vi "LVCAM Msg Receive.vi"(11 "Self Actor in":refnum<class "Self Actor.lvclass">) -> (1 "DeQ Msg?":bool, 2 "Msg":refnum<class "Msg.lvclass">)   [LabVIEW 2021, in "LVCAM.lvlib" / "Self Actor.lvclass"]
uses:
  Self Actor.lvclass
  Msg/Msg.lvclass
  Self Actor.lvclass/Self Actor.ctl
  Msgs/LVCAM Nest Destroyed/LVCAM Nest Destroyed Msg/LVCAM Nest Destroyed Msg.lvclass
  C:/PPLs/LabVIEW-Composed-Actor-Model-LVCAM/LabVIEW-Composed-Actor-Model-LVCAM/AAM/LVCAM/Msg/Msg.lvclass
  Msgs/LVCAM Destroy Self/LVCAM Destroy Self Msg/LVCAM Destroy Self Msg.lvclass
  Msg Q/Msg Q.lvclass
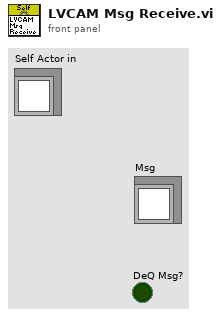
[diagram p1: front panel]
types:
  T1 = typedef "LVCAM.lvlib/Self Actor.lvclass/State.ctl" = enum16{"Safe Msging", "Destroying Self"}
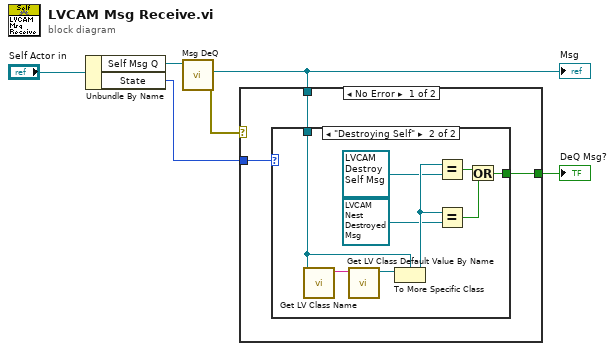
[diagram p0: block diagram]
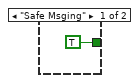
[diagram p2: hidden frame]
diagram:
  n1 = Unbundle By Name("Self Actor in") -> ("Self Msg Q"=w5:refnum<class "Msg Q.lvclass">, "State"=w3:T1)
  n2 = call "Msg DeQ.vi"("Msg Queue in"=w5) -> ("error out"=w6:errorcluster, "Msg"=w1:refnum<class "Msg.lvclass">)  [unwired: 9 in]
  "Msg" <- w1
  n3 = case shown="No Error" w6 {
    tunnel: w1 -> [w7 _]
    tunnel: [w8 _] -> w4
    tunnel: w3 -> [w9 _]
    frame No Error {
      n4 = case shown="\"Destroying Self\"" w9 {
        tunnel: w7 -> [_ w16]
        tunnel: [TRUE w13] -> w8
        frame "Safe Msging" {
        }
        frame "Destroying Self" {
          n5 = call <vilib>:"Get LV Class Name.vi"("object"=w16) -> ("class name"=w19:string)  [unwired: 9 in, 1 out]
          n6 = call <vilib>:"Get LV Class Default Value By Name.vi"("class name"=w19) -> ("object"=w18:refnum<class>)  [unwired: 9 in, 1 out]
          n7 = To More Specific Class(target class=w16, reference=w18) -> (specific class reference=w15:refnum<class "Msg.lvclass">)  [unwired: 1 in, 1 out]
          n8 = Equal?(x=w15, y=refnum<class "LVCAM Destroy Self Msg.lvclass"> refnum ("LVCAM Destroy Self.lvlib:LVCAM Destroy Self Msg.lvclass")) -> (x = y?=w17:bool)
          n9 = Equal?(x=w15, y=refnum<class "LVCAM Nest Destroyed Msg.lvclass"> refnum ("LVCAM Nest Destroyed.lvlib:LVCAM Nest Destroyed Msg.lvclass")) -> (x = y?=w12:bool)
          n10 = Or(x=w17, y=w12) -> (x .or. y?=w13:bool)
        }
      }
    }
    frame Error {
      # "#Handle this error"
    }
  }
  "DeQ Msg?" <- w4
